vi "check test data.vi"(8 "error in":errorcluster, 10 "Array 2":u8[](array[numeric]) format="%x", 11 "Array 1":u8[](array[numeric]) format="%x") -> (0 "error out":errorcluster, 1 "bit numbers":string[](array[string]), 2 "elements 2":u8[](array[numeric]) format="%x", 3 "elements 1":u8[](array[numeric]) format="%x", 4 "total errors":i32, 5 "double errors":i8, 7 "single errors":i8)   [LabVIEW 2017]
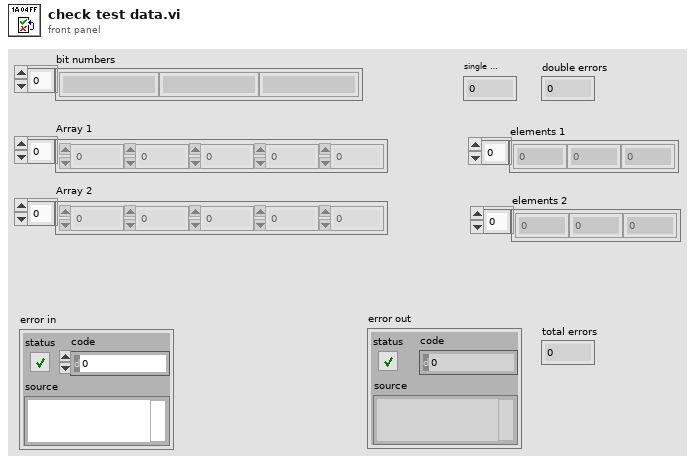
[diagram p1: front panel]
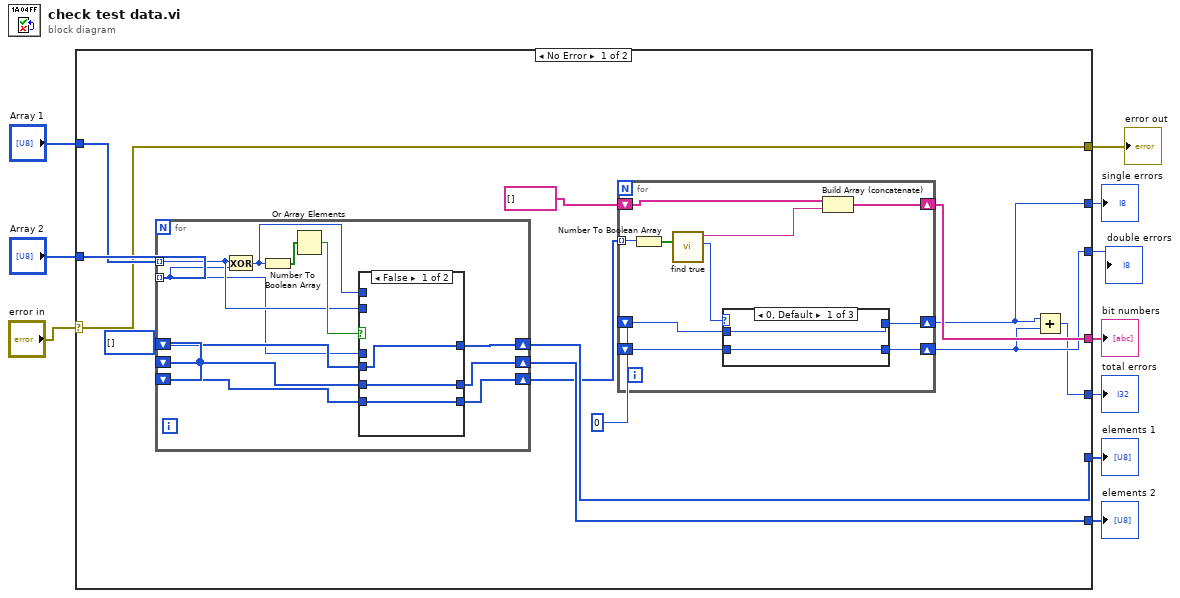
[diagram p0: block diagram]
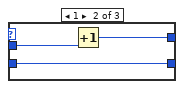
[diagram p2: hidden frame]
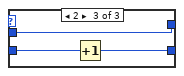
[diagram p3: hidden frame]
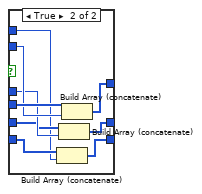
[diagram p4: hidden frame]
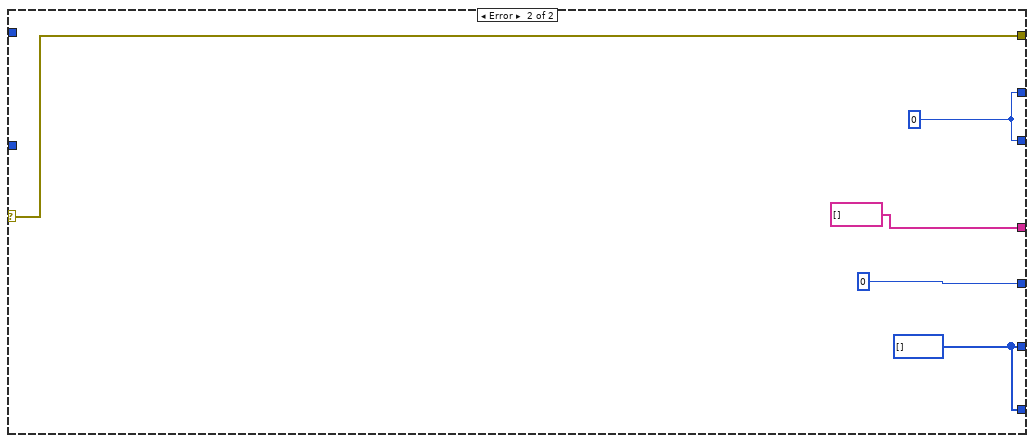
[diagram p5: hidden frame]
diagram:
  n1 = case shown="No Error" "error in" {
    selector: "error in" -> [w20 w69]
    tunnel: [w20 w69] -> w9
    tunnel: "Array 2" -> [w23 _]
    tunnel: "Array 1" -> [w22 _]
    tunnel: [w11 0] -> w6
    tunnel: [w19 w68] -> w5
    tunnel: [w18 w68] -> w4
    tunnel: [w15 string[] []] -> w3
    tunnel: [w13 w65] -> w2
    tunnel: [w12 w65] -> w1
    frame No Error {
      w14 = i8 0
      w21 = u8[] []
      n2 = for {
        tunnel: w23 -> [w44] mode=indexing
        tunnel: w22 -> [w45] mode=indexing
        shift-right: [w42] -> w19
        shift-left: w21 -> [w50]
        shift-right: [w48] -> w18
        shift-left: w21 -> [w49]
        shift-right: [w46] -> w17
        shift-left: w21 -> [w47]
        n3 = Exclusive Or(1:w44, 2:w45) -> (0:w43:u8)
        n4 = Number To Boolean Array(number=w43) -> (Boolean array=w52:bool[])
        n5 = Or Array Elements(Boolean array=w52) -> (logical OR=w51:bool)
        n6 = case shown="False" w51 {
          tunnel: w50 -> [w53 w64]
          tunnel: w49 -> [w55 w60]
          tunnel: [w55 w59] -> w48
          tunnel: w47 -> [w54 w58]
          tunnel: [w54 w56] -> w46
          tunnel: w45 -> [_ w63]
          tunnel: w44 -> [_ w61]
          tunnel: w43 -> [_ w57]
          tunnel: [w53 w62] -> w42
          frame False {
          }
          frame True {
            n7 = Build Array (concatenate)(w58, w57) -> (w56:u8[])
            n8 = Build Array (concatenate)(w60, w61) -> (w59:u8[])
            n9 = Build Array (concatenate)(w64, w63) -> (w62:u8[])
          }
        }
      }
      n10 = for {
        tunnel: w17 -> [w33] mode=indexing
        shift-right: [w29] -> w15
        shift-left: string[] [] -> [w31]
        shift-right: [w24] -> w13
        shift-left: w14 -> [w25]
        shift-right: [w26] -> w12
        shift-left: w14 -> [w27]
        n11 = Number To Boolean Array(number=w33) -> (Boolean array=w32:bool[])
        n12 = call "find true.vi"("Array"=w32) -> ("count"=w28:u8, "numbers"=w30:string)  [unwired: 9 in]
        n13 = case shown="0, Default" w28 {
          tunnel: w27 -> [w35 w38 w41]
          tunnel: [w35 w38 w40] -> w26
          tunnel: w25 -> [w34 w37 w39]
          tunnel: [w34 w36 w39] -> w24
          frame 0, Default {
          }
          frame 1 {
            n14 = Increment(x=w37) -> (x+1=w36:i8)
          }
          frame 2 {
            n15 = Increment(x=w41) -> (x+1=w40:i8)
          }
        }
        n16 = Build Array (concatenate)(w31, w30) -> (w29:string[])
      }
      n17 = Add(x=w13, y=w12) -> (x+y=w11:i8)
    }
    frame Error {
      w65 = i8 0
      w68 = u8[] []
    }
  }
  "error out" <- w9
  "total errors" <- w6
  "elements 1" <- w5
  "elements 2" <- w4
  "bit numbers" <- w3
  "single errors" <- w2
  "double errors" <- w1
